vi "MCL Load Wave Form N.vi"(6 "handle":i32, 7 "waveform":dbl, 9 "milliseconds":dbl, 10 "DataPoints":u32, 11 "axis":u32) -> (3 "function return":i32, 5 "waveform out":dbl)   [LabVIEW 2017, in "Madlib.lvlib"]
doc: "MADLIB_API int MCL_LoadWaveFormN(unsigned int axis,unsigned int DataPoints,double milliseconds,double* waveform, int handle);"
uses:
  Madlib.lvlib
  Madlib.dll
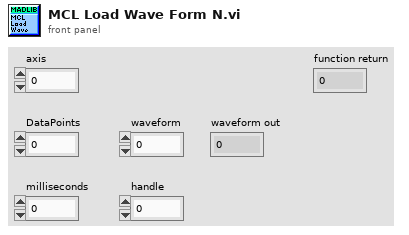
[diagram p1: front panel]
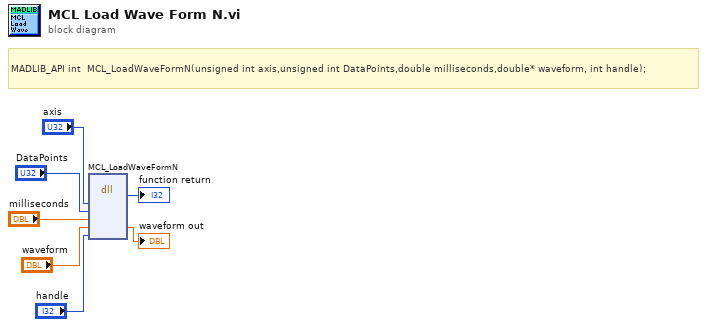
[diagram p0: block diagram]
diagram:
  # "MADLIB_API\tint\t\tMCL_LoadWaveFormN(unsigned int axis,unsigned int DataPoints,double milliseconds,double* waveform, int handle);"
  n1 = dll-call lib="C:/Users/francesco/dev/pump-probe/Piezo/lvlib/Madlib.*" fn="MCL_LoadWaveFormN"("axis"="axis", "DataPoints"="DataPoints", "milliseconds"="milliseconds", "waveform"="waveform", "handle"="handle") -> (→"function return":i32, "waveform"=→"waveform out":dbl)  [unwired: 7 in, 2 out]
